vi "stringHandler.vi"(9 "Data":dbl[](array[numeric]), 10 "Names":string[](array[string])) -> (1 "Input":string, 2 "Header":string)   [LabVIEW 2020]
doc: "This VI takes the logging data and headers and converts it into a format that is readable for the datalogger"
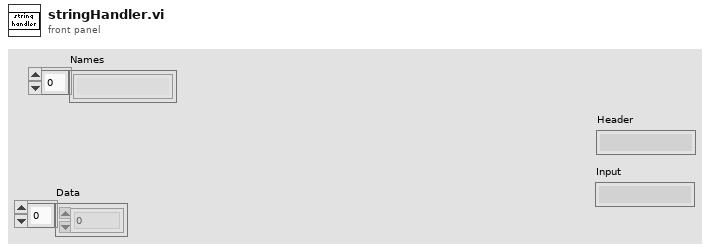
[diagram p1: front panel]
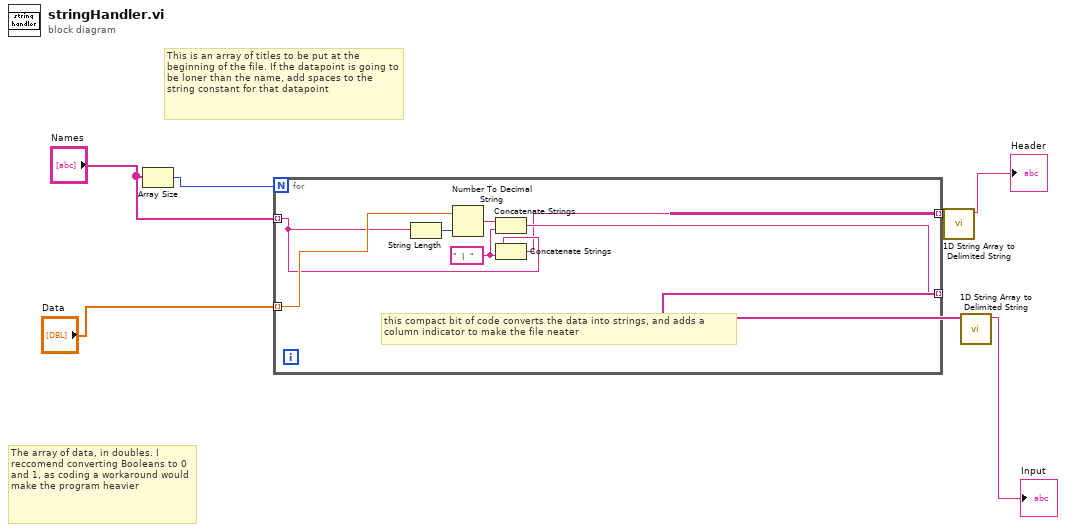
[diagram p0: block diagram]
diagram:
  # "The array of data, in doubles. I reccomend converting Booleans to 0 and 1, as coding a workaround would make the program heavier"
  # "This is an array of titles to be put at the beginning of the file. If the datapoint is going to be loner than the name, add spaces to the string constant for that datapoint"
  n1 = Array Size(array="Names") -> (size(s)=w7:i32)
  n2 = for {
    N: w7 -> [_]
    tunnel: "Names" -> [w12] mode=indexing
    tunnel: "Data" -> [w14] mode=indexing
    tunnel: [w11] -> w2 mode=indexing
    tunnel: [w10] -> w4 mode=indexing
    w8 = "   |   "
    # "this compact bit of code converts the data into strings, and adds a \ncolumn indicator to make the file neater"
    n3 = String Length(string=w12) -> (length=w13:i32)
    n4 = Number To Decimal String(number=w14, width (-)=w13) -> (decimal integer string=w9:string)
    n5 = Concatenate Strings(w9, w8) -> (w11:string)
    n6 = Concatenate Strings(w12, w8) -> (w10:string)
  }
  n7 = call <vilib>:"1D String Array to Delimited String.vi"("string array"=w4) -> ("delimited string"=→"Header":string)  [unwired: 10 in]
  n8 = call <vilib>:"1D String Array to Delimited String.vi"("string array"=w2) -> ("delimited string"=→"Input":string)  [unwired: 10 in]
